vi "Timer Time In Seconds (Reentrant Clone).vi"(7 "Auto Reset?":bool, 9 "milliseconds to wait":u32, 10 "Reset":bool, 11 "Elapsed Time Target [s]":dbl) -> (2 "Time has Elapsed":bool, 3 "Elapsed Time [s]":dbl)   [LabVIEW 2020]
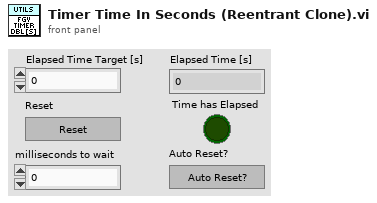
[diagram p1: front panel]
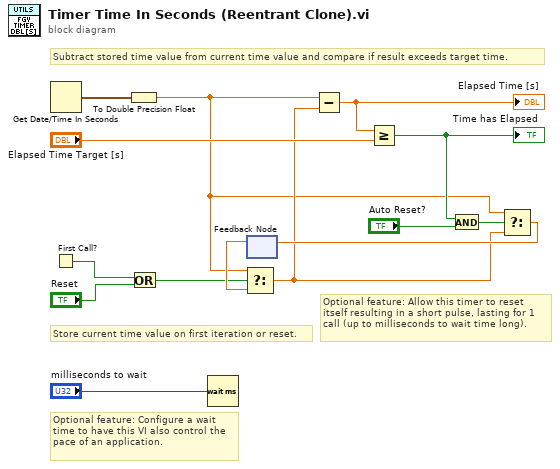
[diagram p0: block diagram]
diagram:
  # "Optional feature: Configure a wait time to have this VI also control the pace of an application."
  # "Optional feature: Allow this timer to reset itself resulting in a short pulse, lasting for 1 call (up to milliseconds to wait time long)."
  # "Store current time value on first iteration or reset."
  # "Subtract stored time value from current time value and compare if result exceeds target time."
  n1 = Get Date/Time In Seconds() -> (seconds since 1Jan1904=w10:timestamp)
  n2 = First Call?() -> (First Call?: T/F=w14:bool)
  n3 = To Double Precision Float(number=w10) -> (double precision float=w2:dbl)
  n4 = Or(x=w14, y="Reset") -> (x .or. y?=w9:bool)
  n5 = Wait (ms)(milliseconds to wait="milliseconds to wait") -> ()  [unwired: 1 out]
  n6 = feedback #1() -> (w13:dbl)  [unwired: 1 in]
  n7 = Select(t=w2, s=w9, f=w13) -> (s? t:f=w3:dbl)
  n8 = Subtract(x=w2, y=w3) -> (x-y=w12:dbl)
  "Elapsed Time [s]" <- w12
  n9 = Greater Or Equal?(x=w12, y="Elapsed Time Target [s]") -> (x >= y?=w8:bool)
  "Time has Elapsed" <- w8
  n10 = And(x=w8, y="Auto Reset?") -> (x .and. y?=w5:bool)
  n11 = Select(t=w2, s=w5, f=w3) -> (s? t:f=w11:dbl)
  n12 = feedback-in #1(w11) -> ()
